vi "Data Format.vi"(9 "Table":refnum<vi>) -> (0 "title":string[](array[string]), 2 "Data":string[](array[string]))   [LabVIEW 2017]
panel:
  out "Error_Description":string
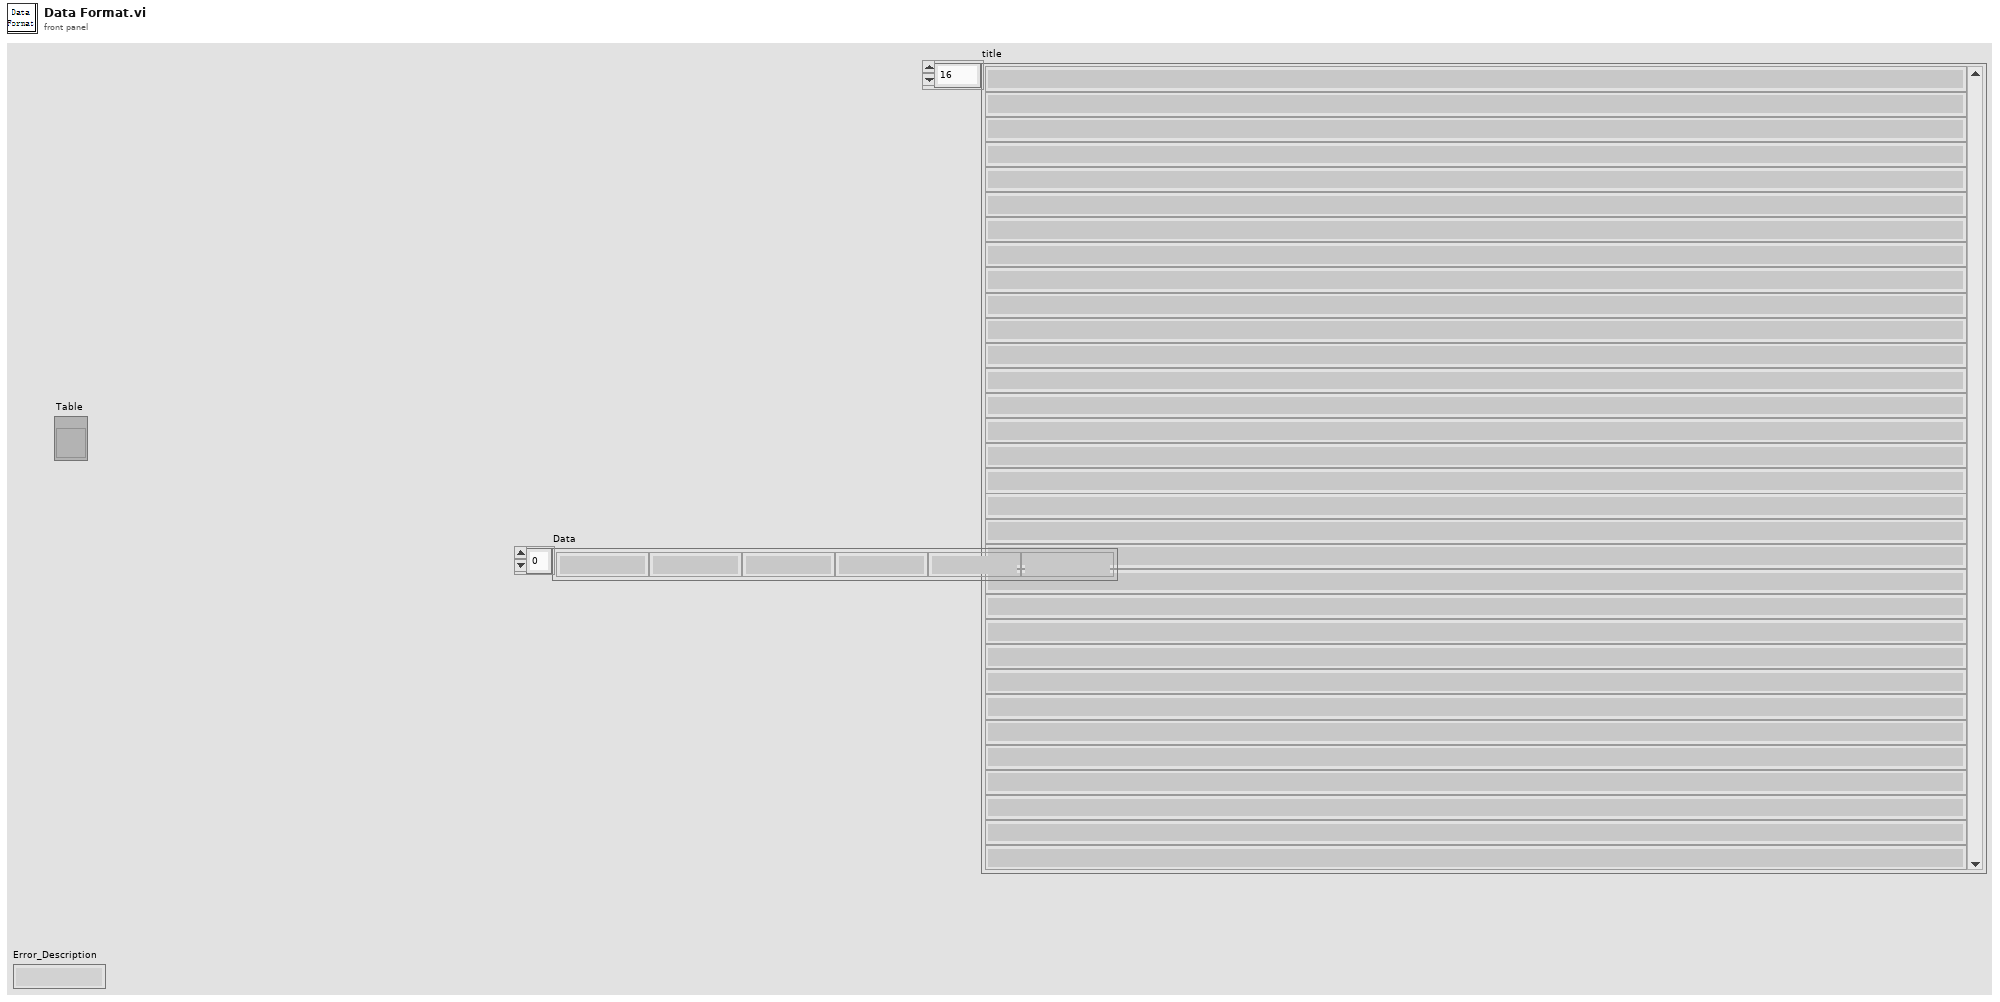
[diagram p1: front panel]
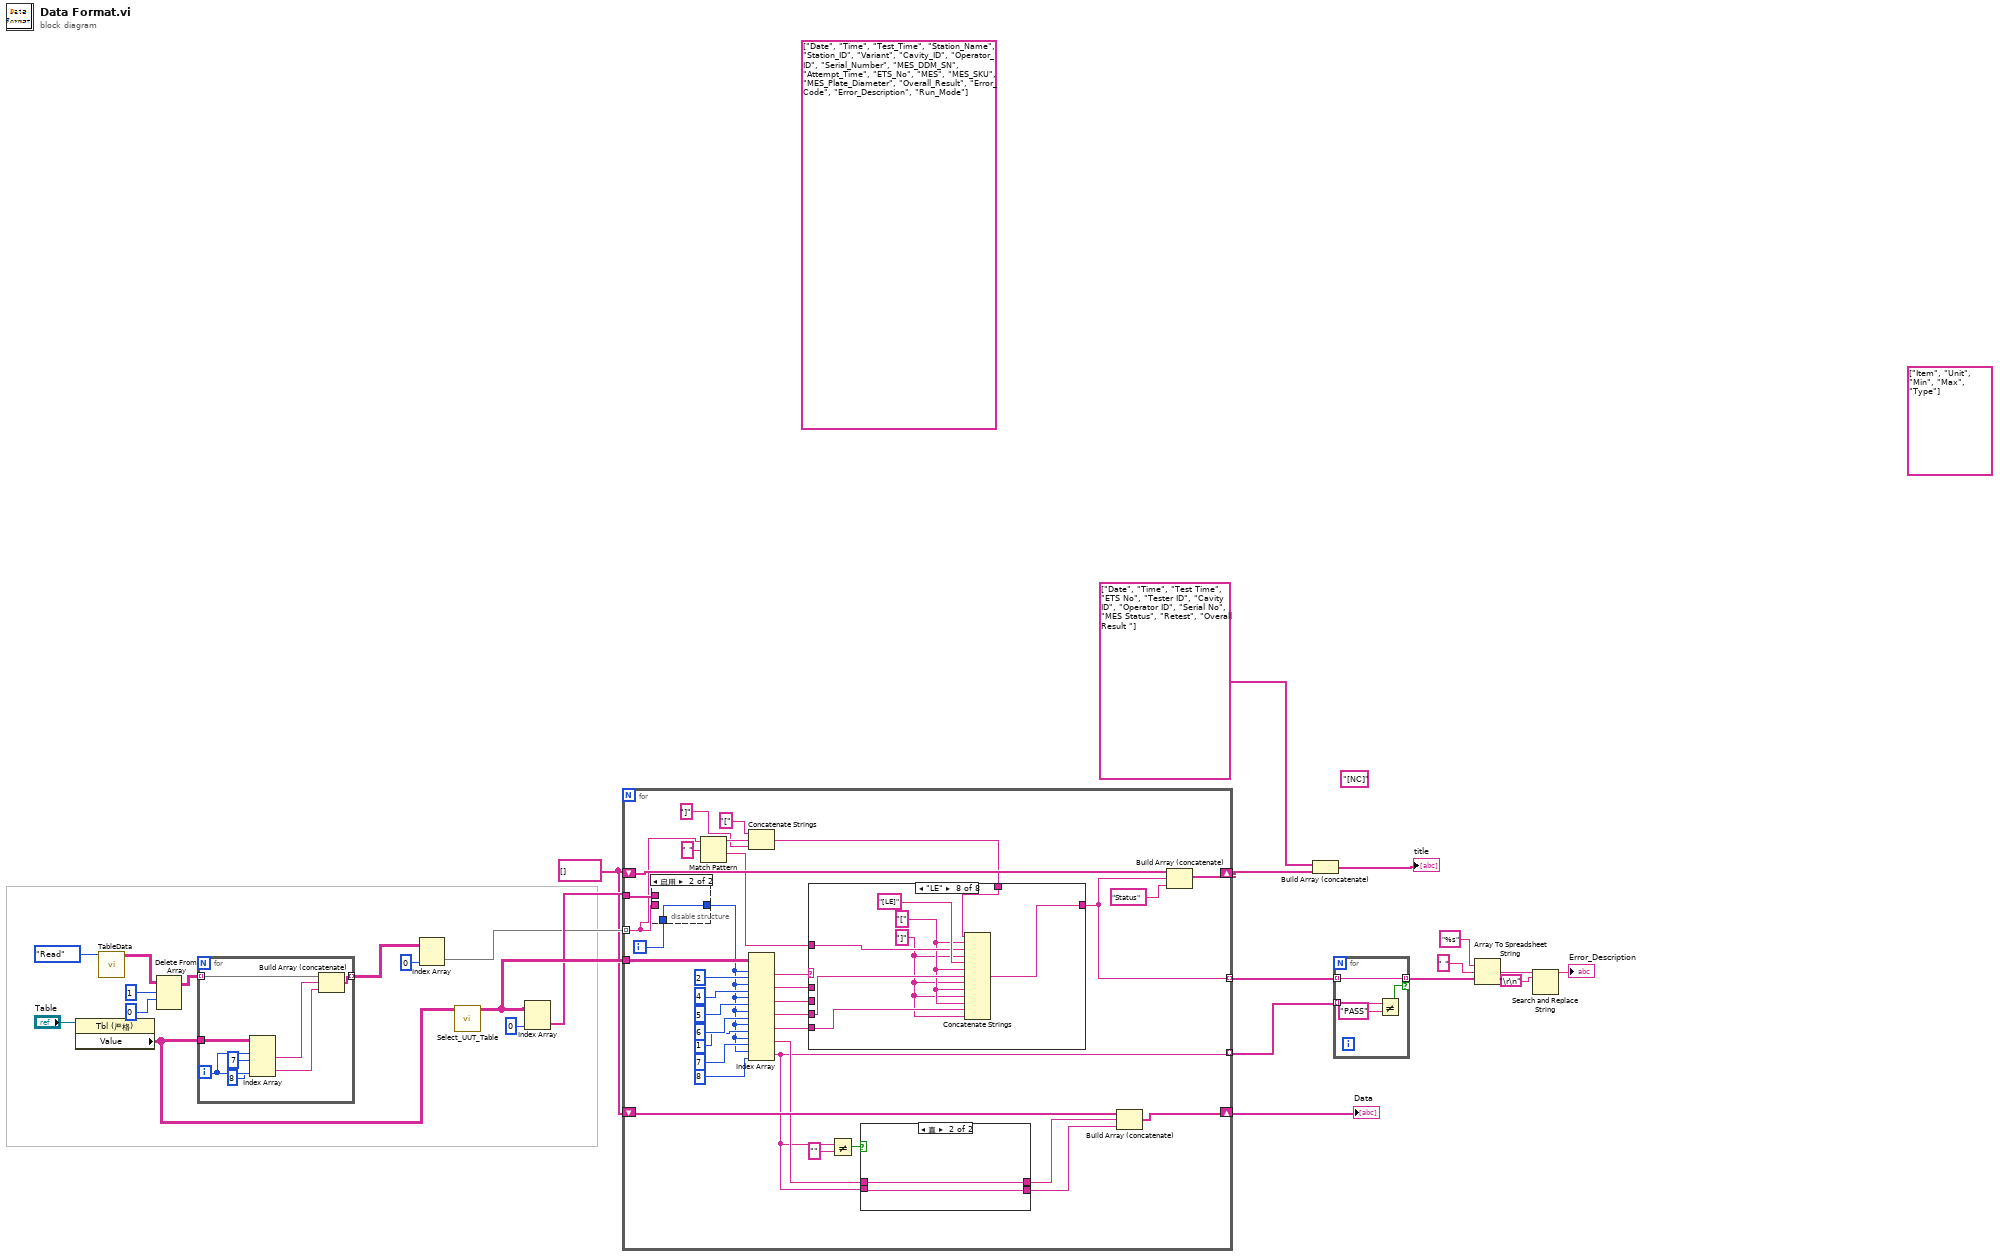
[diagram p0: block diagram]
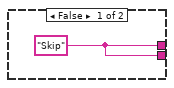
[diagram p2: hidden frame]
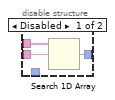
[diagram p3: hidden frame]
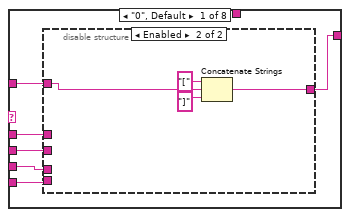
[diagram p4: hidden frame]
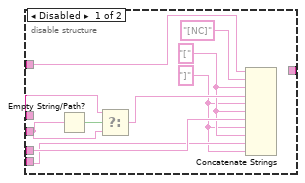
[diagram p5: hidden frame]
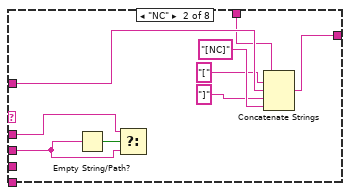
[diagram p6: hidden frame]
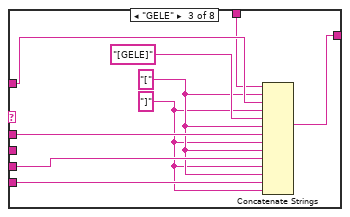
[diagram p7: hidden frame]
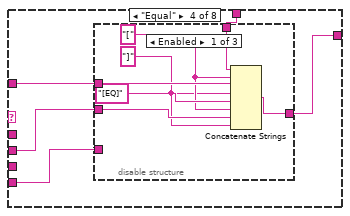
[diagram p8: hidden frame]
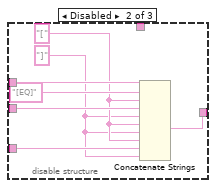
[diagram p9: hidden frame]
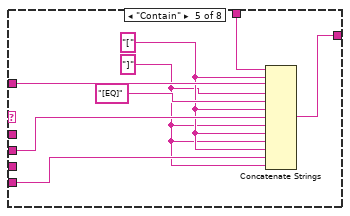
[diagram p11: hidden frame]
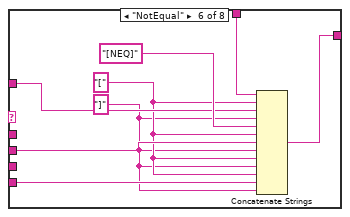
[diagram p12: hidden frame]
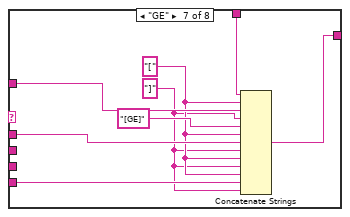
[diagram p13: hidden frame]
diagram:
  (unwired) "[NC]"
  w20 = string[] []
  (unwired) string[] ["Item", "Unit", "Min", "Max", "Type"] ("列首字符串[]")
  (unwired) string[] ["Date", "Time", "Test_Time", "Station_Name", "Station_ID", "Variant", "Cavity_ID", "Operator_ID", "Serial_Number", "MES_DDM_SN", "Attempt_Time", "ETS_No", "MES", "MES_SKU", "MES_Plate_Diameter", "Overall_Result", "Error_Code", "Error_Description", "Run_Mode"]
  n1 = property class="Tbl (严格)"(reference="Table") -> ("Value"=w2:string[][])  [unwired: 1 in, 2 out]
  n2 = call "TableData.vi"("Step"=enum16{"Initial", "Write", "Read"}."Read") -> ("Tabledata Out"=w6:string[][])  [unwired: 9 in, 1 out]
  n3 = Delete From Array(array=w6, length=1, index (row)=0) -> (array with subset deleted=w3:string[][])  [unwired: 1 in, 1 out]
  n4 = for {
    tunnel: w3 -> [w33] mode=indexing
    tunnel: w2 -> [w34]
    tunnel: [w32] -> w7 mode=indexing
    i -> [w31]
    n5 = Index Array(array=w34, index (row) #1=w31, index (col) #1=7 ("index"), index (row) #2=w31, index (col) #2=8 ("index")) -> (element #1=w28:string, element #2=w27:string)
    n6 = Build Array (concatenate)(w33, w28, w27) -> (w32:string[])
  }
  n7 = Index Array "Index Array"(array=w7, index (col)=0 ("禁用的索引 (列)")) -> (element=w21:string[])  [unwired: 1 in]
  n8 = call "Select_UUT_Table.vi"("all Table"=w2) -> ("Table"=w26:string[][])  [unwired: 9 in, 1 out]
  n9 = Index Array(array=w26, index (col)=0 ("禁用的索引 (列)")) -> (element=w24:string[])  [unwired: 1 in]
  n10 = for {
    tunnel: w21 -> [w44] mode=indexing
    tunnel: w26 -> [w68]
    tunnel: w24 -> [w69]
    shift-right: [w58] -> w23
    shift-left: w20 -> [w59]
    shift-right: [w51] -> w19
    shift-left: w20 -> [w52]
    tunnel: [w48] -> w18 mode=indexing
    tunnel: [w37] -> w17 mode=indexing
    i -> [w55]
    n11 = disable-structure shown="启用" {
      disable-tunnel: w69 -> [w75 _]
      disable-tunnel: w44 -> [w74 _]
      disable-tunnel: [w73 w76] -> w50
      disable-tunnel: w55 -> [_ w76]
      frame Disabled {
        n12 = Search 1D Array(1D array=w75, element=w74) -> (index of element=w73:i32)  [unwired: 1 in]
      }
      frame Enabled {
      }
    }
    n13 = Match Pattern(string=w44, regular expression=" ") -> (before substring=w47:string, after substring=w43:string)  [unwired: 1 in, 2 out]
    n14 = Concatenate Strings("[" ("字符串"), w47, "]" ("字符串")) -> (w42:string)
    n15 = Index Array(array=w68, index (row) #1=w50, index (col) #1=2 ("禁用的索引 (列)"), index (row) #2=w50, index (col) #2=4 ("禁用的索引 (列)"), index (row) #3=w50, index (col) #3=5 ("禁用的索引 (列)"), index (row) #4=w50, index (col) #4=6 ("禁用的索引 (列)"), index (row) #5=w50, index (col) #5=1 ("索引 (列)"), index (row) #6=w50, index (col) #6=7 ("disabled index (col)"), index (row) #7=w50, index (col) #7=8 ("disabled index (col)")) -> (element #1=w66:string, element #2=w62:string, element #3=w61:string, element #4=w60:string, element #5=w56:string, element #6=w38:string, element #7=w37:string)
    n16 = case shown="\"LE\"" w66 {
      tunnel: w62 -> [w79 w100 w110 _ _ _ w156 _]
      tunnel: w61 -> [w80 w101 _ w118 w139 w147 _ _]
      tunnel: w60 -> [w82 _ w109 _ _ _ _ w161]
      tunnel: [w77 w103 w112 w117 w138 w146 w154 w163] -> w48
      tunnel: w43 -> [w78 w104 w113 w119 w140 w148 w155 w164]
      tunnel: w56 -> [w81 _ w111 w116 w137 w145 w153 w162]
      tunnel: w42 -> [_ w97 w106 w115 w134 w142 w150 w158]
      frame "0", Default {
        n17 = disable-structure shown="Enabled" {
          disable-tunnel: w82 -> [w91 _]
          disable-tunnel: w81 -> [w90 _]
          disable-tunnel: w80 -> [w88 _]
          disable-tunnel: w79 -> [w87 _]
          disable-tunnel: w78 -> [w83 w96]
          disable-tunnel: [_ w95] -> w77
          frame Disabled {
            w84 = "]" ("字符串")
            w85 = "[" ("字符串")
            n18 = Empty String/Path?(string/path=w88) -> (empty?=w89:bool)
            n19 = Select(t=w87, s=w89, f=w88) -> (s? t:f=w86:string)
            n20 = Concatenate Strings(w83, "[NC]", w85, w86, w84, w85, w91, w84, w85, w90, w84) -> ()  [unwired: 1 out]
          }
          frame Enabled {
            n21 = Concatenate Strings("[" ("string"), w96, "]" ("string")) -> (w95:string)
          }
        }
      }
      frame "NC" {
        n22 = Empty String/Path?(string/path=w101) -> (empty?=w102:bool)
        n23 = Select(t=w100, s=w102, f=w101) -> ()  [unwired: 1 out]
        n24 = Concatenate Strings(w97, "[" ("字符串"), w104, "]" ("字符串"), "[NC]") -> (w103:string)
      }
      frame "GELE" {
        w107 = "]" ("字符串")
        w108 = "[" ("字符串")
        n25 = Concatenate Strings(w106, w108, w113, w107, "[GELE]", w108, w110, w107, w108, w109, w107, w108, w111, w107) -> (w112:string)
      }
      frame "Equal" {
        n26 = disable-structure shown="Enabled" {
          disable-tunnel: w119 -> [w125 w132 _]
          disable-tunnel: w118 -> [w124 w131 _]
          disable-tunnel: [w123 w130 _] -> w117
          disable-tunnel: w116 -> [_ w129 _]
          disable-tunnel: w115 -> [w120 _ _]
          frame Enabled {
            w121 = "]" ("字符串")
            w122 = "[" ("字符串")
            n27 = Concatenate Strings(w120, w122, w125, w121, "[EQ]", w122, w124, w121) -> (w123:string)
          }
          frame Disabled {
            w127 = "]" ("字符串")
            w128 = "[" ("字符串")
            n28 = Concatenate Strings(w132, "[EQ]", w128, w131, w127, w128, w127, w128, w129, w127) -> (w130:string)
          }
          frame Disabled {
          }
        }
      }
      frame "Contain" {
        w135 = "]" ("字符串")
        w136 = "[" ("字符串")
        n29 = Concatenate Strings(w134, w136, w140, w135, "[EQ]", w136, w139, w135, w136, w135, w136, w137, w135) -> (w138:string)
      }
      frame "NotEqual" {
        w143 = "]" ("字符串")
        w144 = "[" ("字符串")
        n30 = Concatenate Strings(w142, w144, w148, w143, "[NEQ]", w144, w147, w143, w144, w143, w144, w145, w143) -> (w146:string)
      }
      frame "GE" {
        w151 = "]" ("字符串")
        w152 = "[" ("字符串")
        n31 = Concatenate Strings(w150, w152, w155, w151, "[GE]", w152, w156, w151, w152, w151, w152, w153, w151) -> (w154:string)
      }
      frame "LE" {
        w159 = "]" ("字符串")
        w160 = "[" ("字符串")
        n32 = Concatenate Strings(w158, w160, w164, w159, "[LE]", w160, w161, w159, w160, w159, w160, w162, w159) -> (w163:string)
      }
    }
    n33 = Not Equal?(x=w37, y="") -> (x != y?=w39:bool)
    n34 = case shown="真" w39 {
      tunnel: w38 -> [_ w72]
      tunnel: [w70 w72] -> w36
      tunnel: [w70 w71] -> w35
      tunnel: w37 -> [_ w71]
      frame False {
        w70 = "Skip" ("y")
      }
      frame True {
      }
    }
    n35 = Build Array (concatenate)(w52, w36, w35) -> (w51:string[])
    n36 = Build Array (concatenate)(w59, w48, "Status" ("element")) -> (w58:string[])
  }
  "Data" <- w19
  n37 = Build Array (concatenate)(string[] ["Date", "Time", "Test Time", "ETS No", "Tester ID", "Cavity ID", "Operator ID", "Serial No", "MES Status", "Retest", "Overall Result "] ("title_beforedata"), w23) -> (→"title":string[])
  n38 = for {
    tunnel: [w169] -> w12 mode=indexing if=w166
    tunnel: w18 -> [w169] mode=indexing
    tunnel: w17 -> [w168] mode=indexing
    n39 = Not Equal?(x=w168, y="PASS") -> (x != y?=w166:bool)
  }
  n40 = Array To Spreadsheet String(delimiter (Tab)=" ", array=w12, 3:"%s" ("delimiter (Tab)")) -> (spreadsheet string=w14:string)
  n41 = Search and Replace String(input string=w14, search string="\r\n") -> (result string=→"Error_Description":string)  [unwired: 6 in, 3 out]
